vi "OVL_Query.vi"(0 "System no.":i32=1 min=1 max=4 step=1, 2 "Channels to query":string[](array[string]), 3 "All channels?":bool, 5 "error in":errorcluster) -> (14 "Velocity":dbl[](array[numeric]) format="%.6f", 19 "error out":errorcluster)   [LabVIEW 2020]
doc: "Returns open-loop velocity in steps/s for specified channels."
panel:
  # "Returns open-loop velocity in steps/s for specified channels."
  # "Query"
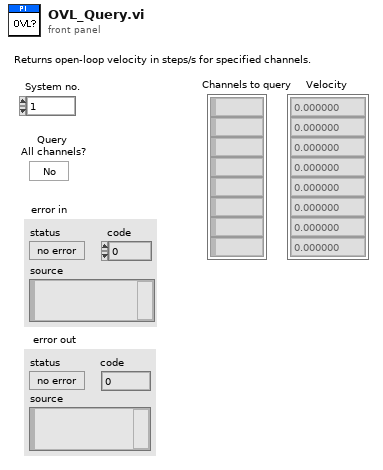
[diagram p1: front panel]
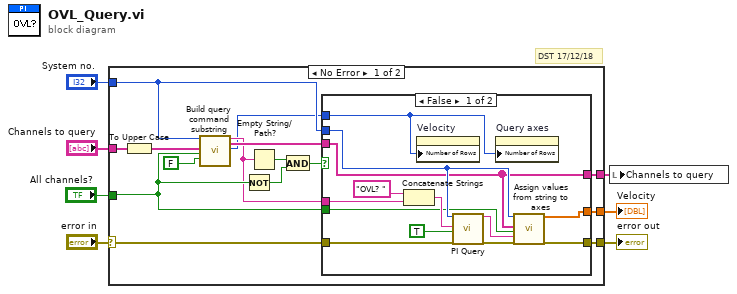
[diagram p0: block diagram]
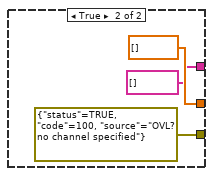
[diagram p2: hidden frame]
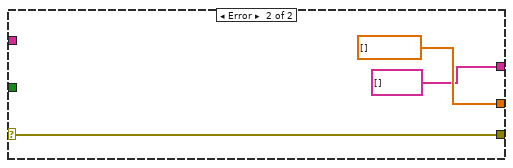
[diagram p3: hidden frame]
diagram:
  # "DST 17/12/18"
  n1 = case shown="No Error" "error in" {
    selector: "error in" -> [w11 w40]
    tunnel: [w22 dbl[] [] ("Values")] -> w7
    tunnel: "Channels to query" -> [w21 _]
    tunnel: [w20 w40] -> w5
    tunnel: "System no." -> [w18 _]
    tunnel: "All channels?" -> [w16 _]
    tunnel: [w8 string[] [] ("Axes to query out")] -> w1
    frame No Error {
      n2 = To Upper Case(1:w21) -> (0:w19:string[])
      n3 = call "Build query command substring.vi"("System no."=w18, "Axes to query in"=w19, "Query\nAll axes?"=w16, "For all axes: use\nAxis identifier?"=FALSE ("For all axes: use\nAxis identifier?")) -> ("Command substring"=w13:string, "Axes to query out"=w17:string[], "Number of rows"=w9:u32)  [unwired: 2 in, 11 out]
      n4 = Not(x=w16) -> (.not. x?=w15:bool)
      n5 = Empty String/Path?(string/path=w13) -> (empty?=w12:bool)
      n6 = And(x=w12, y=w15) -> (x .and. y?=w10:bool)
      n7 = case shown="False" w10 {
        tunnel: [w32 dbl[] [] ("Values")] -> w22
        tunnel: [w29 errorcluster {"status"=TRUE, "code"=100, "source"="OVL? no channel specified"} ("error out")] -> w20
        tunnel: w18 -> [w31 _]
        tunnel: w17 -> [w23 _]
        tunnel: w16 -> [w30 _]
        tunnel: w13 -> [w26 _]
        tunnel: w11 -> [w25 _]
        tunnel: w9 -> [w24 _]
        tunnel: [w23 string[] [] ("Axes to query out")] -> w8
        frame False {
          n8 = Concatenate Strings("OVL? ", w26) -> (w33:string)
          n9 = property on="Velocity" class="Arr (strict)"("Number of Rows"=w24) -> ()  [unwired: 2 in, 2 out]
          n10 = call "PI Query.vi"("System no."=w31, "String to send"=w33, "Attach termination char.?"=TRUE ("Attach Linefeed?"), "error in"=w25) -> ("String read"=w28:string, "error out"=w27:errorcluster)  [unwired: 3 in, 11 out]
          n11 = property on="Query axes" class="Arr (strict)"("Number of Rows"=w24) -> ()  [unwired: 2 in, 2 out]
          n12 = call "Assign values from string to axes.vi"("System no."=w31, "Queried axes"=w23, "All axes queried?"=w30, "Input String"=w28, "error in"=w27) -> ("Values"=w32:dbl[], "error out"=w29:errorcluster)  [unwired: 4 in, 9 out]
        }
        frame True {
        }
      }
    }
    frame Error {
    }
  }
  "error out" <- w5
  "Velocity" <- w7
  n13 = local write "Channels to query"(w1) -> ()
